vi "DAQmx Analog.vi"(8 "error in (no error)":errorcluster, 10 "Analog input #":u8, 11 "DAQmx Analog in":refnum<class "DAQmx Analog.lvclass">) -> (0 "error out":errorcluster, 3 "DAQmx Analog out":refnum<class "DAQmx Analog.lvclass">)   [LabVIEW 2017, in "DAQmx Analog.lvclass"]
uses:
  DAQmx Analog.lvclass
  C:/LabVIEW-programs-dev/Instruments/Utility Classes/Readable/Readable.lvclass
  Utility Classes/Readable/Channel Units.ctl
  DAQmx Analog.lvclass/DAQmx Analog.ctl
  <vilib>/DAQmx/create/channels.llb/DAQmx Create Channel (AI-Voltage-Basic).vi
  <vilib>/DAQmx/configure/timing.llb/DAQmx Timing (Sample Clock).vi
  Utility Classes/Readable/Readable.lvclass
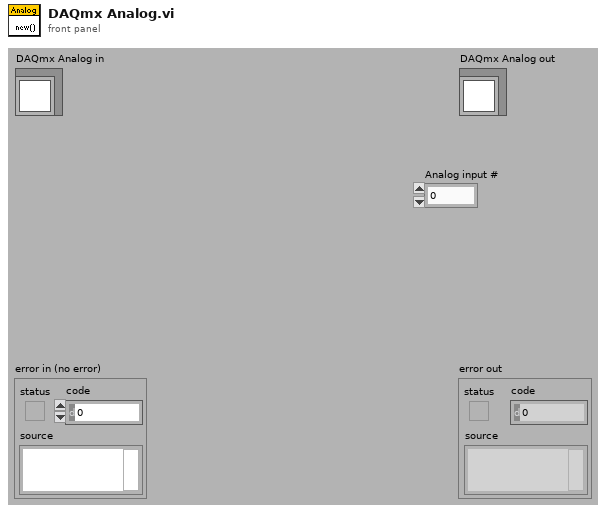
[diagram p1: front panel]
types:
  T1 = typedef "Readable.lvclass/Channel Units.ctl" = string[]
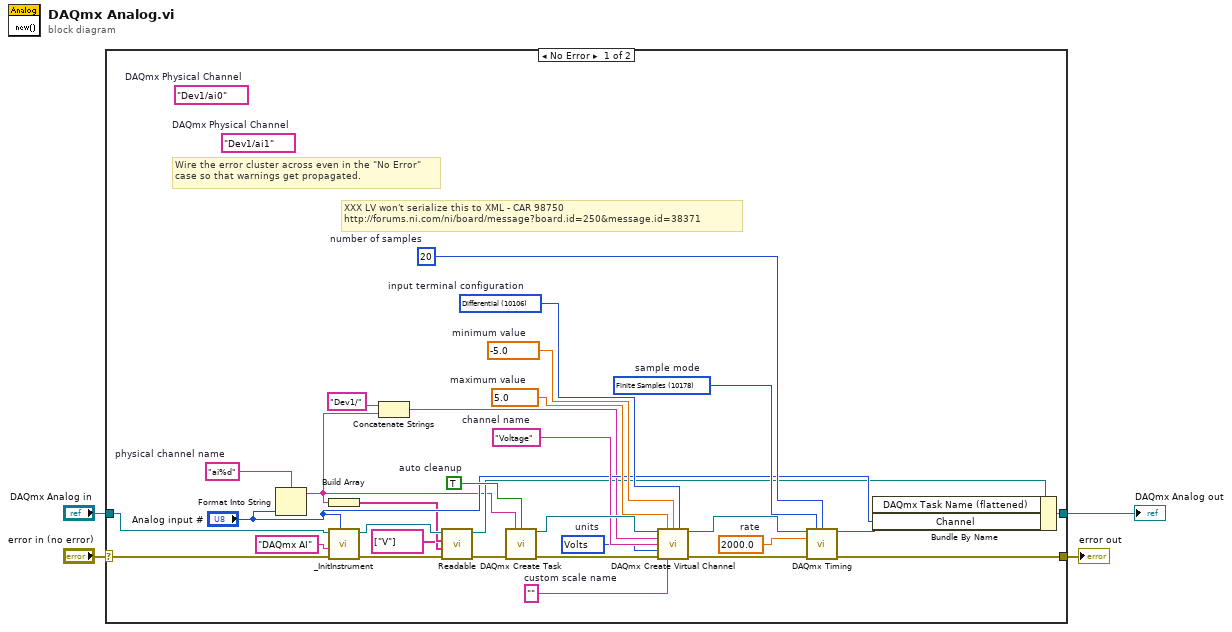
[diagram p0: block diagram]
diagram:
  n1 = case shown="No Error" "error in (no error)" {
    selector: "error in (no error)" -> [w19 w37]
    tunnel: [w15 w37] -> w3
    tunnel: [w21 w36] -> w1
    tunnel: "DAQmx Analog in" -> [w17 w36]
    frame No Error {
      w24 = 2000.0  # rate
      w29 = -5.0  # minimum value
      w30 = 5.0  # maximum value
      w14 = "ai%d"  # physical channel name
      (unwired) tag "Dev1/ai1"  # DAQmx Physical Channel
      (unwired) tag "Dev1/ai0"  # DAQmx Physical Channel
      w22 = 10178 items=["Finite Samples"=10178, "Continuous Samples"=10123, "Hardware Timed Single Point"=12522]  # sample mode
      w23 = 20  # number of samples
      w25 = 10106 items=["default"=-1, "RSE"=10083, "NRSE"=10078, "Differential"=10106, "Pseudodifferential"=12529]  # input terminal configuration
      w26 = 10348 items=["Volts"=10348, "From Custom Scale"=10065]  # units
      w27 = "Voltage"  # channel name
      w28 = ""  # custom scale name
      w32 = TRUE  # auto cleanup
      # "XXX LV won't serialize this to XML - CAR 98750 \nhttp://forums.ni.com/ni/board/message?board.id=250&message.id=38371"
      # "Wire the error cluster across even in the \"No Error\"\ncase so that warnings get propagated."
      n2 = Format Into String(format string=w14, "Analog input #") -> (resulting string=w7:string)  [unwired: 2 in, 1 out]
      n3 = Build Array(w7) -> (w6:string[])
      n4 = call-dynamic "_InitInstrument.vi"("Channel"="Analog input #", "error in (no error)"=w19, "Name"="DAQmx AI", "Instrument in"=w17) -> ("error out"=w9:errorcluster, "Instrument out"=w18:refnum<class "DAQmx Analog.lvclass">)  [unwired: 2 in, 4 out]
      n5 = Concatenate Strings("Dev1/" ("string"), w7) -> (w11:string)
      n6 = call "Readable.vi"("error in (no error)"=w9, "Channel Units"=T1 ["V"], "Channel Names"=w6, "Readable in"=w18) -> ("error out"=w8:errorcluster, "Readable out"=w10:refnum<class "DAQmx Analog.lvclass">)  [unwired: 6 in]
      n7 = call <vilib>:"DAQmx Create Task.vi"("new task name"=w7, "auto cleanup"=w32, "error in"=w8) -> ("task out"=w31:refnum<k21>, "error out"=w33:errorcluster)  [unwired: 2 in, 9 out]
      n8 = call-poly <vilib>:"DAQmx Create Virtual Channel.vi"("task in"=w31, "maximum value"=w30, "minimum value"=w29, "input terminal configuration"=w25, "physical channels"=w11, "name to assign"=w27, "units"=w26, "error in"=w33, "custom scale name"=w28) -> ("task out"=w34:refnum<k21>, "error out"=w35:errorcluster)  [unwired: 5 out]
      n9 = call-poly <vilib>:"DAQmx Timing.vi"("task/channels in"=w34, "sample mode"=w22, "samples per channel"=w23, "rate"=w24, "error in"=w35) -> ("task out"=w16:refnum<k21>, "error out"=w15:errorcluster)  [unwired: 2 in, 7 out]
      n10 = Bundle By Name(cluster=w10, "DAQmx Task Name (flattened)"=w16, "Channel"="Analog input #") -> (w21:refnum<class "DAQmx Analog.lvclass">)
    }
    frame Error {
    }
  }
  "error out" <- w3
  "DAQmx Analog out" <- w1
